vi "STFT_Example.vi"() -> ()   [LabVIEW 2014]
uses:
  <vilib>/Analysis/3filter.llb/Filter Passband Type.ctl
  <vilib>/Analysis/4window.llb/windowTd.ctl
  <vilib>/Utility/file.llb/Read From Spreadsheet File (DBL).vi
  <vilib>/Analysis/3filter.llb/Butterworth Filter (DBL).vi
  <vilib>/Analysis/NI_AALBase.lvlib
  <vilib>/gmath/NI_Gmath.lvlib
  <vilib>/Analysis/NI_AALPro.lvlib
panel:
  out "STFT Spectrogram {X}":dbl[][](array[numeric])
  in  "stop":bool
  out "EEG":dbl[][](graph)
  in  "Trial Number":i32=1
  in  "Frame_Length":i32=20
  in  "Flash_Repeat":i32=20
  in  "Random_num":i32=6
  in  "EEG Data":path
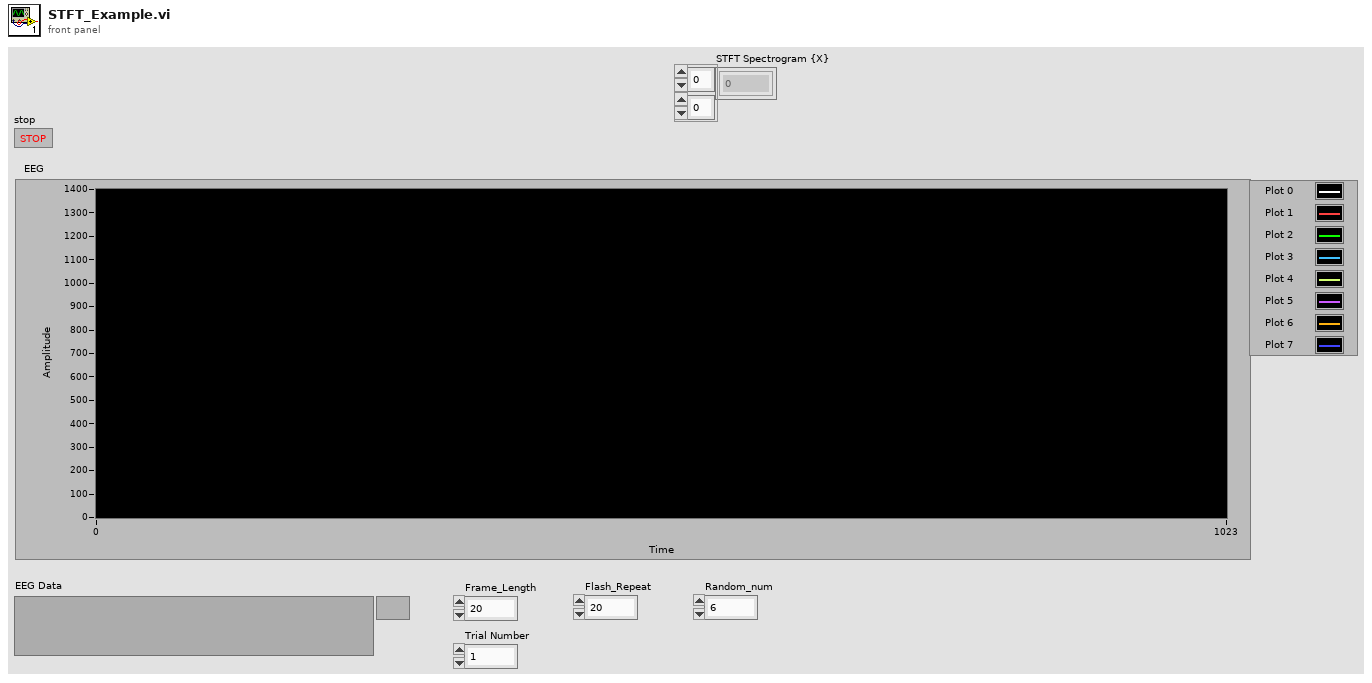
[diagram p1: front panel]
types:
  T1 = typedef "NI_AALPro.lvlib/windowTd.ctl" = u32
  T2 = typedef "NI_AALBase.lvlib/Filter Passband Type.ctl" = enum32{"Lowpass", "Highpass", "Bandpass", "Bandstop"}
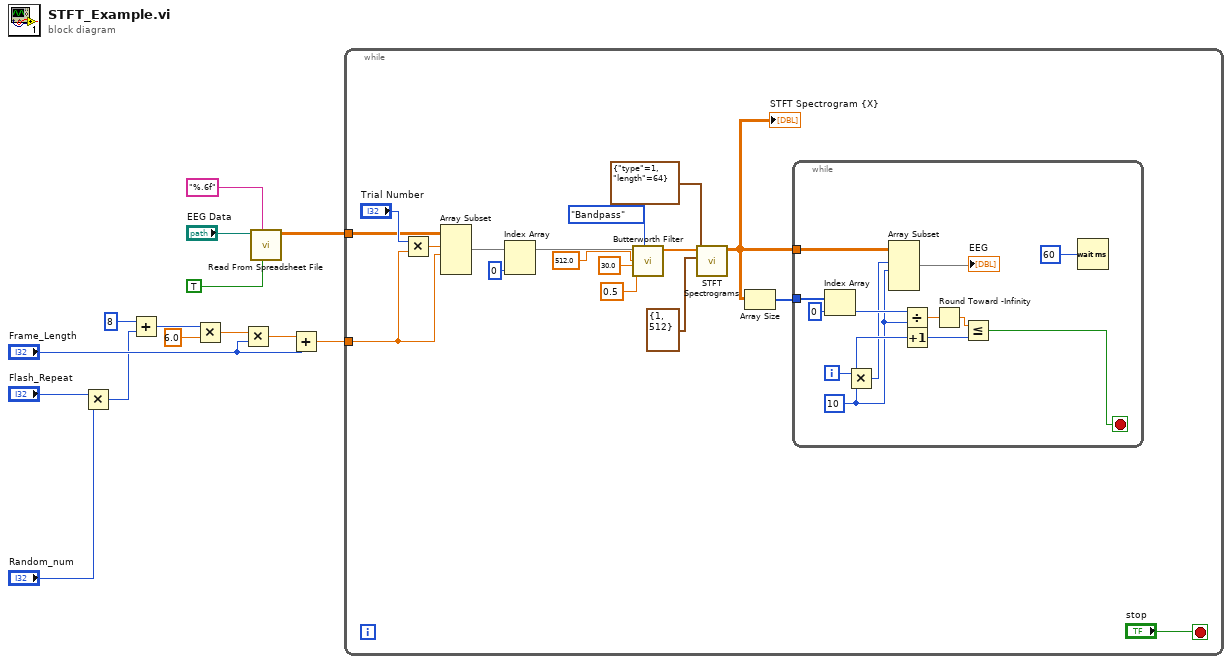
[diagram p0: block diagram]
diagram:
  n1 = Multiply(x="Flash_Repeat", y="Random_num") -> (x*y=w7:i32)
  n2 = Add(x=8, y=w7) -> (x+y=w5:i32)
  n3 = Multiply(x=w5, y=6.0) -> (x*y=w3:dbl)
  n4 = Multiply(x=w3, y="Frame_Length") -> (x*y=w2:dbl)
  n5 = call-poly <vilib>:"Read From Spreadsheet File.vi"("transpose (no:F)"=TRUE, "format (%.3f)"="%.6f", "file path (dialog if empty)"="EEG Data") -> ("all rows"=w11:dbl[][])  [unwired: 4 in, 4 out]
  n6 = Add(x=w2, y="Frame_Length") -> (x+y=w1:dbl)
  n7 = while {
    tunnel: w11 -> [w24]
    tunnel: w1 -> [w23]
    stop <- "stop" stop-if-true
    n8 = Multiply(x="Trial Number", y=w23) -> (x*y=w25:dbl)
    n9 = Array Subset(array=w24, index (row)=w25, length (row)=w23) -> (w22:dbl[][])  [unwired: 2 in]
    n10 = Index Array(array=w22, index (col)=0 ("disabled index (col)")) -> (element=w19:dbl[])  [unwired: 1 in]
    n11 = call-poly <vilib>:"Butterworth Filter.vi"("filter type"=Filter_Passband_Type."Bandpass", "low cutoff freq: fl"=0.5, "high cutoff freq: fh"=30.0, "sampling freq: fs"=512.0 ("high cutoff freq: fh"), "X"=w19) -> ("Filtered X"=w18:dbl[])  [unwired: 3 in, 1 out]
    n12 = call <vilib>:"STFT Spectrograms.vi"("window info"=cluster{"type":T1, "length":i32} {"type"=1, "length"=64}, "time-freq sampling info"=cluster{"time steps":i32, "frequency bins":i32} {"time steps"=1, "frequency bins"=512}, "X"=w18) -> ("STFT Spectrogram {X}"=w15:dbl[][])  [unwired: 7 in, 1 out]
    "STFT Spectrogram {X}" <- w15
    n13 = Array Size(array=w15) -> (size(s)=w21:i32[])
    n14 = while {
      tunnel: w15 -> [w44]
      tunnel: w21 -> [w40]
      i -> [w37]
      stop <- w36 stop-if-true
      w32 = 10
      n15 = Index Array(array=w40, index=0) -> (element=w38:i32)
      n16 = Multiply(x=w37, y=w32) -> (x*y=w33:i32)
      n17 = Array Subset(array=w44, index (row)=w33, length (row)=w32) -> (→"EEG":dbl[][])  [unwired: 2 in]
      n18 = Divide(x=w38, y=w32) -> (x/y=w42:dbl)
      n19 = Increment(x=w37) -> (x+1=w43:i32)
      n20 = Round Toward -Infinity(1:w42) -> (0:w41:dbl)
      n21 = Less Or Equal?(x=w41, y=w43) -> (x <= y?=w36:bool)
      n22 = Wait (ms)(milliseconds to wait=u32 60) -> ()  [unwired: 1 out]
    }
  }
